vi "Image.Num to Color, Grey_Yellow_Green_Red.vi"(11 "Num":i32) -> (3 "Color":u32(colorbox))   [LabVIEW 2018]
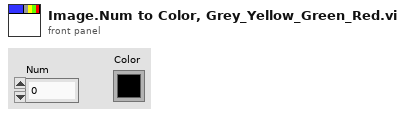
[diagram p1: front panel]
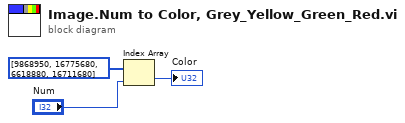
[diagram p0: block diagram]
diagram:
  n1 = Index Array(array=u32[] [9868950, 16775680, 6618880, 16711680], index="Num") -> (element=→"Color":u32)
